vi "Remove All Aliases.vi"(8 "error in":errorcluster, 11 "aliases in":T1 format="%.0x") -> (0 "error out":errorcluster, 3 "aliases out":T1 format="%.0x")   [LabVIEW 2020, in "Routing and Faulting Scripting.lvlib"]
doc: "Removes all aliases from the custom device."
uses:
  Routing and Faulting Scripting.lvlib
  <vilib>/NI VeriStand/Custom Device API/Custom Device Item Ref.ctl
  <vilib>/NI VeriStand/Custom Device API/Custom Device API.lvlib
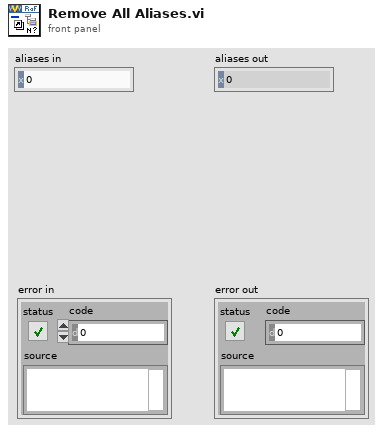
[diagram p1: front panel]
types:
  T1 = typedef "Custom Device API.lvlib/Custom Device Item Ref.ctl" = u64
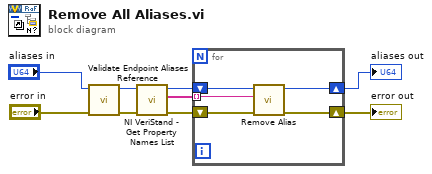
[diagram p0: block diagram]
diagram:
  n1 = call "Validate Endpoint Aliases Reference.vi"("error in"="error in", "endpoint aliases in"="aliases in") -> ("error out"=w3:errorcluster, "endpoint aliases out"=w1:T1)  [unwired: 8 in]
  n2 = call <vilib>:"NI VeriStand - Get Property Names List.vi"("error in (no error)"=w3, "Item Ref in"=w1) -> ("error out"=w8:errorcluster, "Property Names"=w9:string[], "Item Ref out"=w5:T1)  [unwired: 7 in]
  n3 = for {
    tunnel: w9 -> [w12] mode=indexing
    shift-right: [w10] -> w6
    shift-left: w8 -> [w11]
    shift-right: [w13] -> w4
    shift-left: w5 -> [w14]
    n4 = call "Remove Alias.vi"("error in"=w11, "alias"=w12, "endpoint aliases in"=w14) -> ("error out"=w10:errorcluster, "endpoint aliases out"=w13:T1)  [unwired: 7 in]
  }
  "error out" <- w6
  "aliases out" <- w4
